vi "Generate Subject Strings.vi"(3 "Number of Subjects":i32) -> (1 "Array":string[](array[string]))   [LabVIEW 2019]
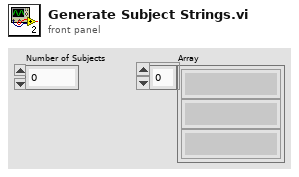
[diagram p1: front panel]
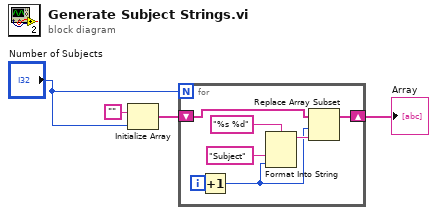
[diagram p0: block diagram]
diagram:
  n1 = Initialize Array("", "Number of Subjects") -> (w1:string[])
  n2 = for {
    N: "Number of Subjects" -> [_]
    shift-right: [w7] -> w3
    shift-left: w1 -> [w11]
    i -> [w8]
    n3 = Increment(x=w8) -> (x+1=w5:i32)
    n4 = Format Into String(format string="%s %d", "Subject" ("input 1"), w5) -> (resulting string=w6:string)  [unwired: 2 in, 1 out]
    n5 = Replace Array Subset(array=w11, new element=w6, index=w5) -> (w7:string[])
  }
  "Array" <- w3
